vi "delta.vi"(8 "error in (no error)":errorcluster, 11 "KNR in":T1) -> (0 "error out":errorcluster, 3 "KNR out":T1)   [LabVIEW 2013]
uses:
  <userlib>/KNR OS 3.0 LabVIEW Toolkit/Type Definition/KNR3 Reference.ctl
  <userlib>/_FPGA Interface Advanced Tools/FPGA Interface Base/FPGA Interface Base.lvclass
  <userlib>/KNR OS 3.0 LabVIEW Toolkit/Type Definition/Resource.ctl
  Global 1.vi
panel:
  in  "STOP 2":bool
  in  "left 2":bool
  in  "right 2":bool
  in  "STOP":bool
  in  "left":bool
  in  "right":bool
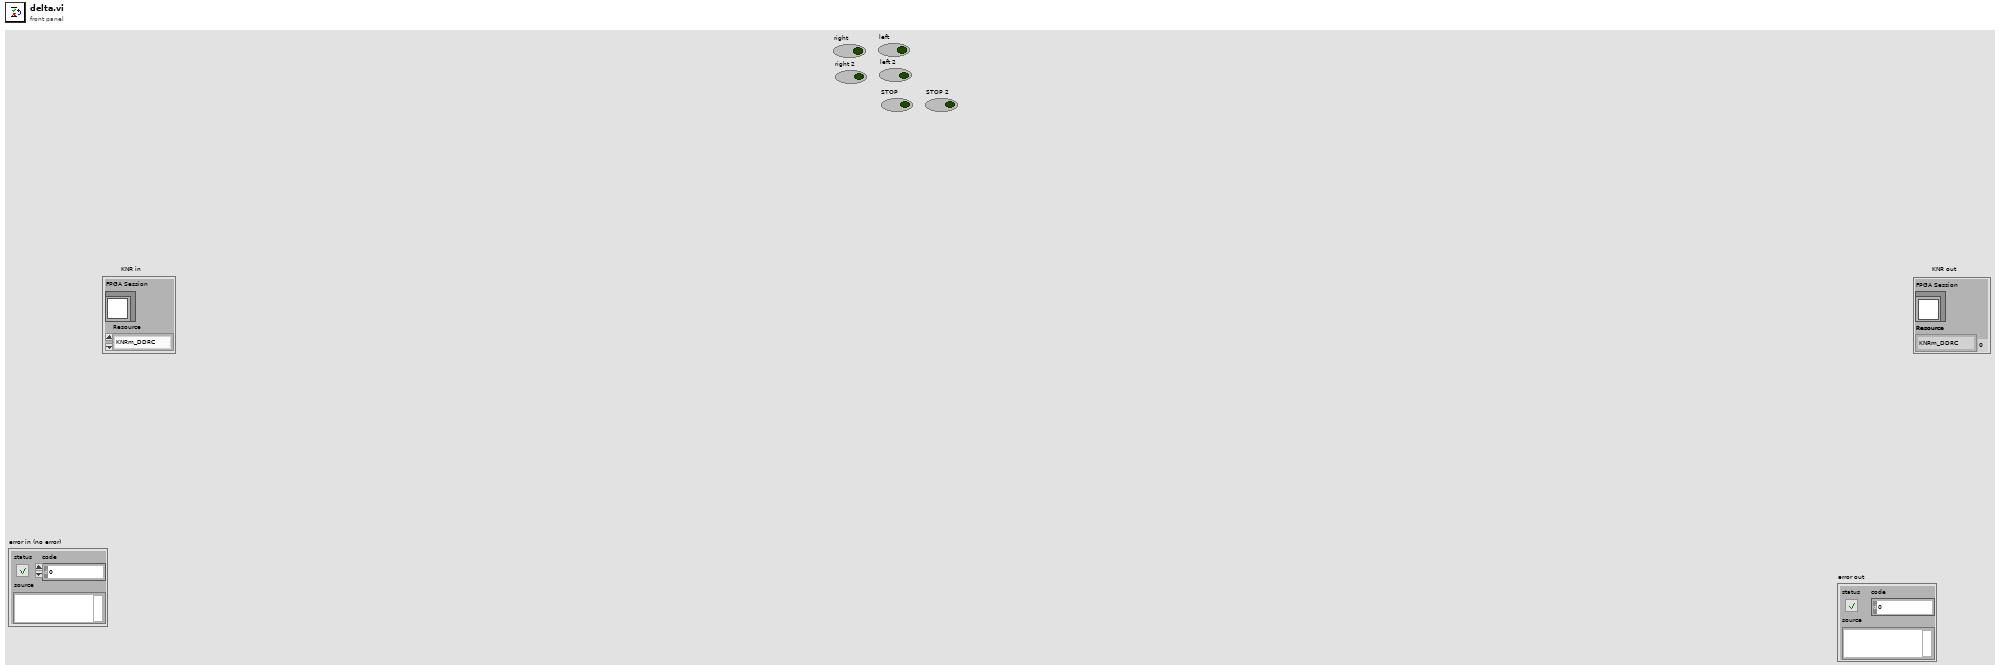
[diagram p1: front panel]
types:
  T1 = typedef "KNR3 Reference.ctl" = cluster{"FPGA Session":refnum<class "FPGA Interface Base.lvclass">, "Resource":T2}
  T2 = typedef "Resource.ctl" = enum16{"KNRm_DDRC", "KNRm_DDDD", "KNRm_DDDR", "KNRm_DDDC", "KNR"}
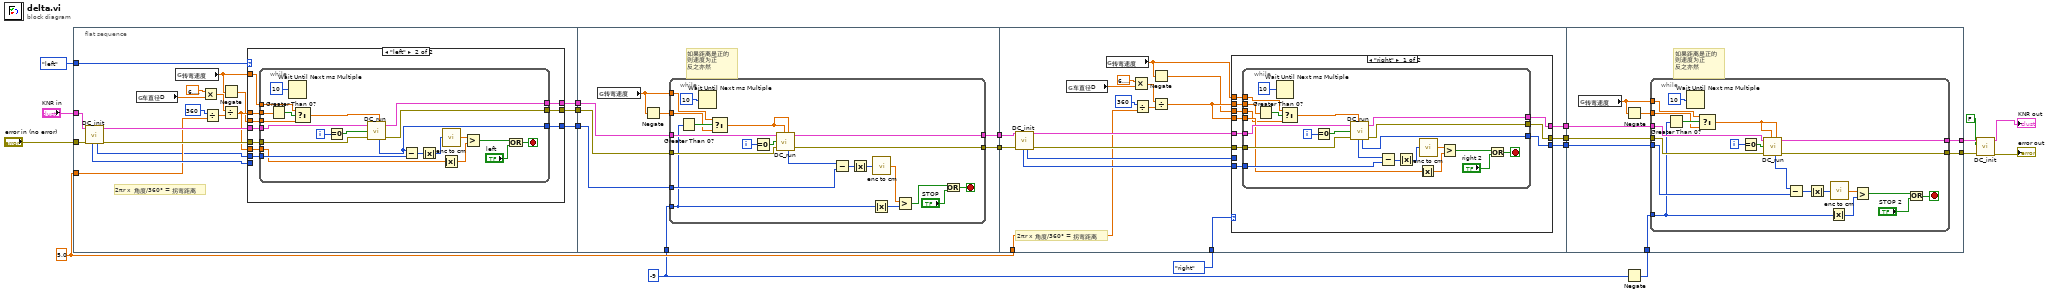
[diagram p0: block diagram]
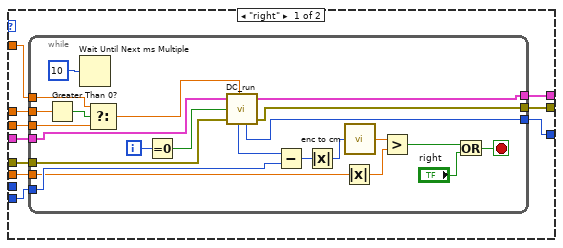
[diagram p2: hidden frame]
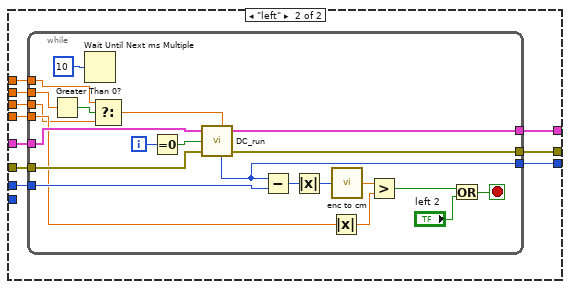
[diagram p3: hidden frame]
diagram:
  w14 = 5.0
  w10 = -9
  n1 = flat-sequence {
    tunnel: "KNR in" -> [w28]
    tunnel: "error in (no error)" -> [w27]
    tunnel: enum16{"right", "left"}."left" -> [w26]
    tunnel: w14 -> [w25]
    tunnel: [w23] -> w18
    tunnel: [w22] -> w17
    tunnel: [w21] -> w16
    tunnel: w18 -> [w110]
    tunnel: w17 -> [w109]
    tunnel: w16 -> [w108]
    tunnel: w10 -> [w107]
    tunnel: [w106] -> w12
    tunnel: [w105] -> w11
    tunnel: enum16{"right", "left"}."right" -> [w140]
    tunnel: w14 -> [w139]
    tunnel: w12 -> [w138]
    tunnel: w11 -> [w137]
    tunnel: [w136] -> w8
    tunnel: [w135] -> w7
    tunnel: [w134] -> w6
    tunnel: w9 -> [w223]
    tunnel: w8 -> [w222]
    tunnel: w7 -> [w221]
    tunnel: w6 -> [w220]
    tunnel: [w219] -> w5
    tunnel: [w218] -> w4
    frame #0 {
      # "2πr x 角度/360° = 拐弯距离"
      n2 = call "DC_init.vi"("error in (no error)"=w27, "KNR in"=w28) -> ("error out"=w34:errorcluster, "KNR out"=w35:T1, "output\nposition 2"=w24:i32, "output\nPosition_1"=w32:i32)  [unwired: 6 in]
      n3 = global read "Global 1.vi" "车直径D"() -> (w31:dbl)
      n4 = global read "Global 1.vi" "转弯速度"() -> (w29:dbl)
      n5 = Multiply(x=6.283185307179586, y=w31) -> (x*y=w37:dbl)
      n6 = Divide(x=360, y=w25) -> (x/y=w36:dbl)
      n7 = Negate(x=w29) -> (-x=w30:dbl)
      n8 = Divide(x=w37, y=w36) -> (x/y=w33:dbl)
      n9 = case shown="\"left\"" w26 {
        tunnel: w33 -> [w49 w80]
        tunnel: [w48 w79] -> w23
        tunnel: [w47 w78] -> w22
        tunnel: w35 -> [w46 w81]
        tunnel: w34 -> [w45 w82]
        tunnel: w24 -> [_ w77]
        tunnel: w33 -> [w43 w76]
        tunnel: w32 -> [w44 _]
        tunnel: w29 -> [w42 w75]
        tunnel: w30 -> [w41 w74]
        tunnel: [w40 w73] -> w21
        frame "right" {
          n10 = while {
            tunnel: w49 -> [w57]
            tunnel: w46 -> [w70]
            tunnel: w45 -> [w69]
            tunnel: [w61] -> w48
            tunnel: [w60] -> w47
            tunnel: w44 -> [w58]
            tunnel: w43 -> [w55]
            tunnel: w42 -> [w52]
            tunnel: w41 -> [w51]
            tunnel: [w50] -> w40
            i -> [w68]
            stop <- w59 stop-if-true
            n11 = Greater Than 0?(x=w57) -> (x > 0?=w72:bool)
            n12 = Wait Until Next ms Multiple(millisecond multiple=u32 10) -> ()  [unwired: 1 out]
            n13 = Select(t=w52, s=w72, f=w51) -> (s? t:f=w62:dbl)
            n14 = Equal To 0?(x=w68) -> (x = 0?=w67:bool)
            n15 = call "DC_run.vi"("KNR in"=w70, "speed_1"=w62, "reinitialize? (F)"=w67, "error in (no error)"=w69) -> ("Position_1"=w54:i32, "KNR out"=w61:T1, "Position_2"=w50:i32, "error out"=w60:errorcluster)  [unwired: 2 in]
            n16 = Subtract(x=w54, y=w58) -> (x-y=w66:i32)
            n17 = Absolute Value(x=w66) -> (abs(x)=w63:i32)
            n18 = Absolute Value(x=w55) -> (abs(x)=w65:dbl)
            n19 = call "enc to cm.vi"("E"=w63) -> ("CM"=w53:dbl)  [unwired: 1 in]
            n20 = Greater?(x=w53, y=w65) -> (0:w64:bool)
            n21 = Or(x=w64, y="right") -> (x .or. y?=w59:bool)
          }
        }
        frame "left" {
          n22 = while {
            tunnel: w80 -> [w89]
            tunnel: w81 -> [w102]
            tunnel: w82 -> [w101]
            tunnel: [w93] -> w79
            tunnel: [w92] -> w78
            tunnel: w77 -> [w90]
            tunnel: w76 -> [w87]
            tunnel: w75 -> [w85]
            tunnel: w74 -> [w84]
            tunnel: [w83] -> w73
            i -> [w100]
            stop <- w94 stop-if-true
            n23 = Greater Than 0?(x=w89) -> (x > 0?=w104:bool)
            n24 = Wait Until Next ms Multiple(millisecond multiple=u32 10) -> ()  [unwired: 1 out]
            n25 = Select(t=w85, s=w104, f=w84) -> (s? t:f=w91:dbl)
            n26 = Equal To 0?(x=w100) -> (x = 0?=w99:bool)
            n27 = call "DC_run.vi"("KNR in"=w102, "reinitialize? (F)"=w99, "error in (no error)"=w101, "speed_2"=w91) -> ("KNR out"=w93:T1, "Position_2"=w83:i32, "error out"=w92:errorcluster)  [unwired: 2 in, 1 out]
            n28 = Subtract(x=w83, y=w90) -> (x-y=w98:i32)
            n29 = Absolute Value(x=w98) -> (abs(x)=w95:i32)
            n30 = Absolute Value(x=w87) -> (abs(x)=w97:dbl)
            n31 = call "enc to cm.vi"("E"=w95) -> ("CM"=w86:dbl)  [unwired: 1 in]
            n32 = Greater?(x=w86, y=w97) -> (0:w96:bool)
            n33 = Or(x=w96, y="left") -> (x .or. y?=w94:bool)
          }
        }
      }
    }
    frame #1 {
      # "如果距离是正的\n则速度为正\n反之亦然"
      n34 = global read "Global 1.vi" "转弯速度"() -> (w111:dbl)
      n35 = Negate(x=w111) -> (-x=w112:dbl)
      n36 = while {
        tunnel: w110 -> [w131]
        tunnel: w109 -> [w130]
        tunnel: [w122] -> w106
        tunnel: [w121] -> w105
        tunnel: w108 -> [w118]
        tunnel: w107 -> [w117]
        tunnel: w111 -> [w116]
        tunnel: w112 -> [w115]
        i -> [w127]
        stop <- w113 stop-if-true
        n37 = Greater Than 0?(x=w117) -> (x > 0?=w132:bool)
        n38 = Wait Until Next ms Multiple(millisecond multiple=u32 10) -> ()  [unwired: 1 out]
        n39 = Select(t=w116, s=w132, f=w115) -> (s? t:f=w129:dbl)
        n40 = Equal To 0?(x=w127) -> (x = 0?=w128:bool)
        n41 = call "DC_run.vi"("KNR in"=w131, "speed_1"=w129, "reinitialize? (F)"=w128, "error in (no error)"=w130, "speed_2"=w129) -> ("KNR out"=w122:T1, "Position_2"=w119:i32, "error out"=w121:errorcluster)  [unwired: 1 in, 1 out]
        n42 = Subtract(x=w119, y=w118) -> (x-y=w126:i32)
        n43 = Absolute Value(x=w126) -> (abs(x)=w123:i32)
        n44 = Absolute Value(x=w117) -> (abs(x)=w125:i32)
        n45 = call "enc to cm.vi"("E"=w123) -> ("CM"=w120:dbl)  [unwired: 1 in]
        n46 = Greater?(x=w120, y=w125) -> (0:w124:bool)
        n47 = Or(x=w124, y="STOP") -> (x .or. y?=w113:bool)
      }
    }
    frame #2 {
      # "2πr x 角度/360° = 拐弯距离"
      n48 = call "DC_init.vi"("error in (no error)"=w137, "KNR in"=w138) -> ("error out"=w147:errorcluster, "KNR out"=w148:T1, "output\nposition 2"=w141:i32, "output\nPosition_1"=w145:i32)  [unwired: 6 in]
      n49 = global read "Global 1.vi" "车直径D"() -> (w144:dbl)
      n50 = global read "Global 1.vi" "转弯速度"() -> (w142:dbl)
      n51 = Multiply(x=6.283185307179586, y=w144) -> (x*y=w150:dbl)
      n52 = Divide(x=360, y=w139) -> (x/y=w149:dbl)
      n53 = Negate(x=w142) -> (-x=w143:dbl)
      n54 = Divide(x=w150, y=w149) -> (x/y=w146:dbl)
      n55 = case shown="\"right\"" w140 {
        tunnel: w146 -> [w162 w193]
        tunnel: [w161 w192] -> w136
        tunnel: [w160 w191] -> w135
        tunnel: w148 -> [w159 w194]
        tunnel: w147 -> [w158 w195]
        tunnel: w141 -> [_ w190]
        tunnel: w146 -> [w156 w189]
        tunnel: w145 -> [w157 _]
        tunnel: w142 -> [w155 w188]
        tunnel: w143 -> [w154 w187]
        tunnel: [w153 w186] -> w134
        frame "right" {
          n56 = while {
            tunnel: w162 -> [w170]
            tunnel: w159 -> [w183]
            tunnel: w158 -> [w182]
            tunnel: [w174] -> w161
            tunnel: [w173] -> w160
            tunnel: w157 -> [w171]
            tunnel: w156 -> [w168]
            tunnel: w155 -> [w165]
            tunnel: w154 -> [w164]
            tunnel: [w163] -> w153
            i -> [w181]
            stop <- w172 stop-if-true
            n57 = Greater Than 0?(x=w170) -> (x > 0?=w185:bool)
            n58 = Wait Until Next ms Multiple(millisecond multiple=u32 10) -> ()  [unwired: 1 out]
            n59 = Select(t=w165, s=w185, f=w164) -> (s? t:f=w175:dbl)
            n60 = Equal To 0?(x=w181) -> (x = 0?=w180:bool)
            n61 = call "DC_run.vi"("KNR in"=w183, "speed_1"=w175, "reinitialize? (F)"=w180, "error in (no error)"=w182) -> ("Position_1"=w167:i32, "KNR out"=w174:T1, "Position_2"=w163:i32, "error out"=w173:errorcluster)  [unwired: 2 in]
            n62 = Subtract(x=w167, y=w171) -> (x-y=w179:i32)
            n63 = Absolute Value(x=w179) -> (abs(x)=w176:i32)
            n64 = Absolute Value(x=w168) -> (abs(x)=w178:dbl)
            n65 = call "enc to cm.vi"("E"=w176) -> ("CM"=w166:dbl)  [unwired: 1 in]
            n66 = Greater?(x=w166, y=w178) -> (0:w177:bool)
            n67 = Or(x=w177, y="right 2") -> (x .or. y?=w172:bool)
          }
        }
        frame "left" {
          n68 = while {
            tunnel: w193 -> [w202]
            tunnel: w194 -> [w215]
            tunnel: w195 -> [w214]
            tunnel: [w206] -> w192
            tunnel: [w205] -> w191
            tunnel: w190 -> [w203]
            tunnel: w189 -> [w200]
            tunnel: w188 -> [w198]
            tunnel: w187 -> [w197]
            tunnel: [w196] -> w186
            i -> [w213]
            stop <- w207 stop-if-true
            n69 = Greater Than 0?(x=w202) -> (x > 0?=w217:bool)
            n70 = Wait Until Next ms Multiple(millisecond multiple=u32 10) -> ()  [unwired: 1 out]
            n71 = Select(t=w198, s=w217, f=w197) -> (s? t:f=w204:dbl)
            n72 = Equal To 0?(x=w213) -> (x = 0?=w212:bool)
            n73 = call "DC_run.vi"("KNR in"=w215, "reinitialize? (F)"=w212, "error in (no error)"=w214, "speed_2"=w204) -> ("KNR out"=w206:T1, "Position_2"=w196:i32, "error out"=w205:errorcluster)  [unwired: 2 in, 1 out]
            n74 = Subtract(x=w196, y=w203) -> (x-y=w211:i32)
            n75 = Absolute Value(x=w211) -> (abs(x)=w208:i32)
            n76 = Absolute Value(x=w200) -> (abs(x)=w210:dbl)
            n77 = call "enc to cm.vi"("E"=w208) -> ("CM"=w199:dbl)  [unwired: 1 in]
            n78 = Greater?(x=w199, y=w210) -> (0:w209:bool)
            n79 = Or(x=w209, y="left 2") -> (x .or. y?=w207:bool)
          }
        }
      }
    }
    frame #3 {
      # "如果距离是正的\n则速度为正\n反之亦然"
      n80 = global read "Global 1.vi" "转弯速度"() -> (w224:dbl)
      n81 = Negate(x=w224) -> (-x=w225:dbl)
      n82 = while {
        tunnel: w222 -> [w244]
        tunnel: w221 -> [w243]
        tunnel: [w235] -> w218
        tunnel: [w234] -> w219
        tunnel: w220 -> [w231]
        tunnel: w223 -> [w230]
        tunnel: w224 -> [w229]
        tunnel: w225 -> [w228]
        i -> [w240]
        stop <- w226 stop-if-true
        n83 = Greater Than 0?(x=w230) -> (x > 0?=w245:bool)
        n84 = Wait Until Next ms Multiple(millisecond multiple=u32 10) -> ()  [unwired: 1 out]
        n85 = Select(t=w229, s=w245, f=w228) -> (s? t:f=w242:dbl)
        n86 = Equal To 0?(x=w240) -> (x = 0?=w241:bool)
        n87 = call "DC_run.vi"("KNR in"=w244, "speed_1"=w242, "reinitialize? (F)"=w241, "error in (no error)"=w243, "speed_2"=w242) -> ("KNR out"=w235:T1, "Position_2"=w232:i32, "error out"=w234:errorcluster)  [unwired: 1 in, 1 out]
        n88 = Subtract(x=w232, y=w231) -> (x-y=w239:i32)
        n89 = Absolute Value(x=w239) -> (abs(x)=w236:i32)
        n90 = Absolute Value(x=w230) -> (abs(x)=w238:i32)
        n91 = call "enc to cm.vi"("E"=w236) -> ("CM"=w233:dbl)  [unwired: 1 in]
        n92 = Greater?(x=w233, y=w238) -> (0:w237:bool)
        n93 = Or(x=w237, y="STOP 2") -> (x .or. y?=w226:bool)
      }
    }
  }
  n94 = Negate(x=w10) -> (-x=w9:i32)
  n95 = call "DC_init.vi"("error in (no error)"=w5, "Enable Motor(T)"=FALSE, "KNR in"=w4) -> ("error out"=→"error out":errorcluster, "KNR out"=→"KNR out":T1)  [unwired: 5 in, 2 out]
